vi "getSparaConfig.vi"(0 "Spec Associate":string[][](table), 5 "different":string[](array[string]), 9 "smooth":bool[](array[boolean]), 11 "XML document":path caption="XML文档路径", 12 "smoothPoints":dbl=1.0 min=1.0 max=100.0 step=2.0) -> (4 "sPara":T1[](array[typedef]), 6 "extPara":T1[](array[typedef]))   [LabVIEW 2011]
uses:
  dataType/singleTestParameter.ctl
panel:
  out "extParaSmooth":bool[](array[boolean])
  out "sParaSmooth":bool[](array[boolean])
  in  "spec 2":T2
  in  "spec":T2
  out "namelist":string[](array[string])
  out "valueArray":string[][](array[string])
  out "extPara":string[](array[string])
  out "sPara":string[](array[string])
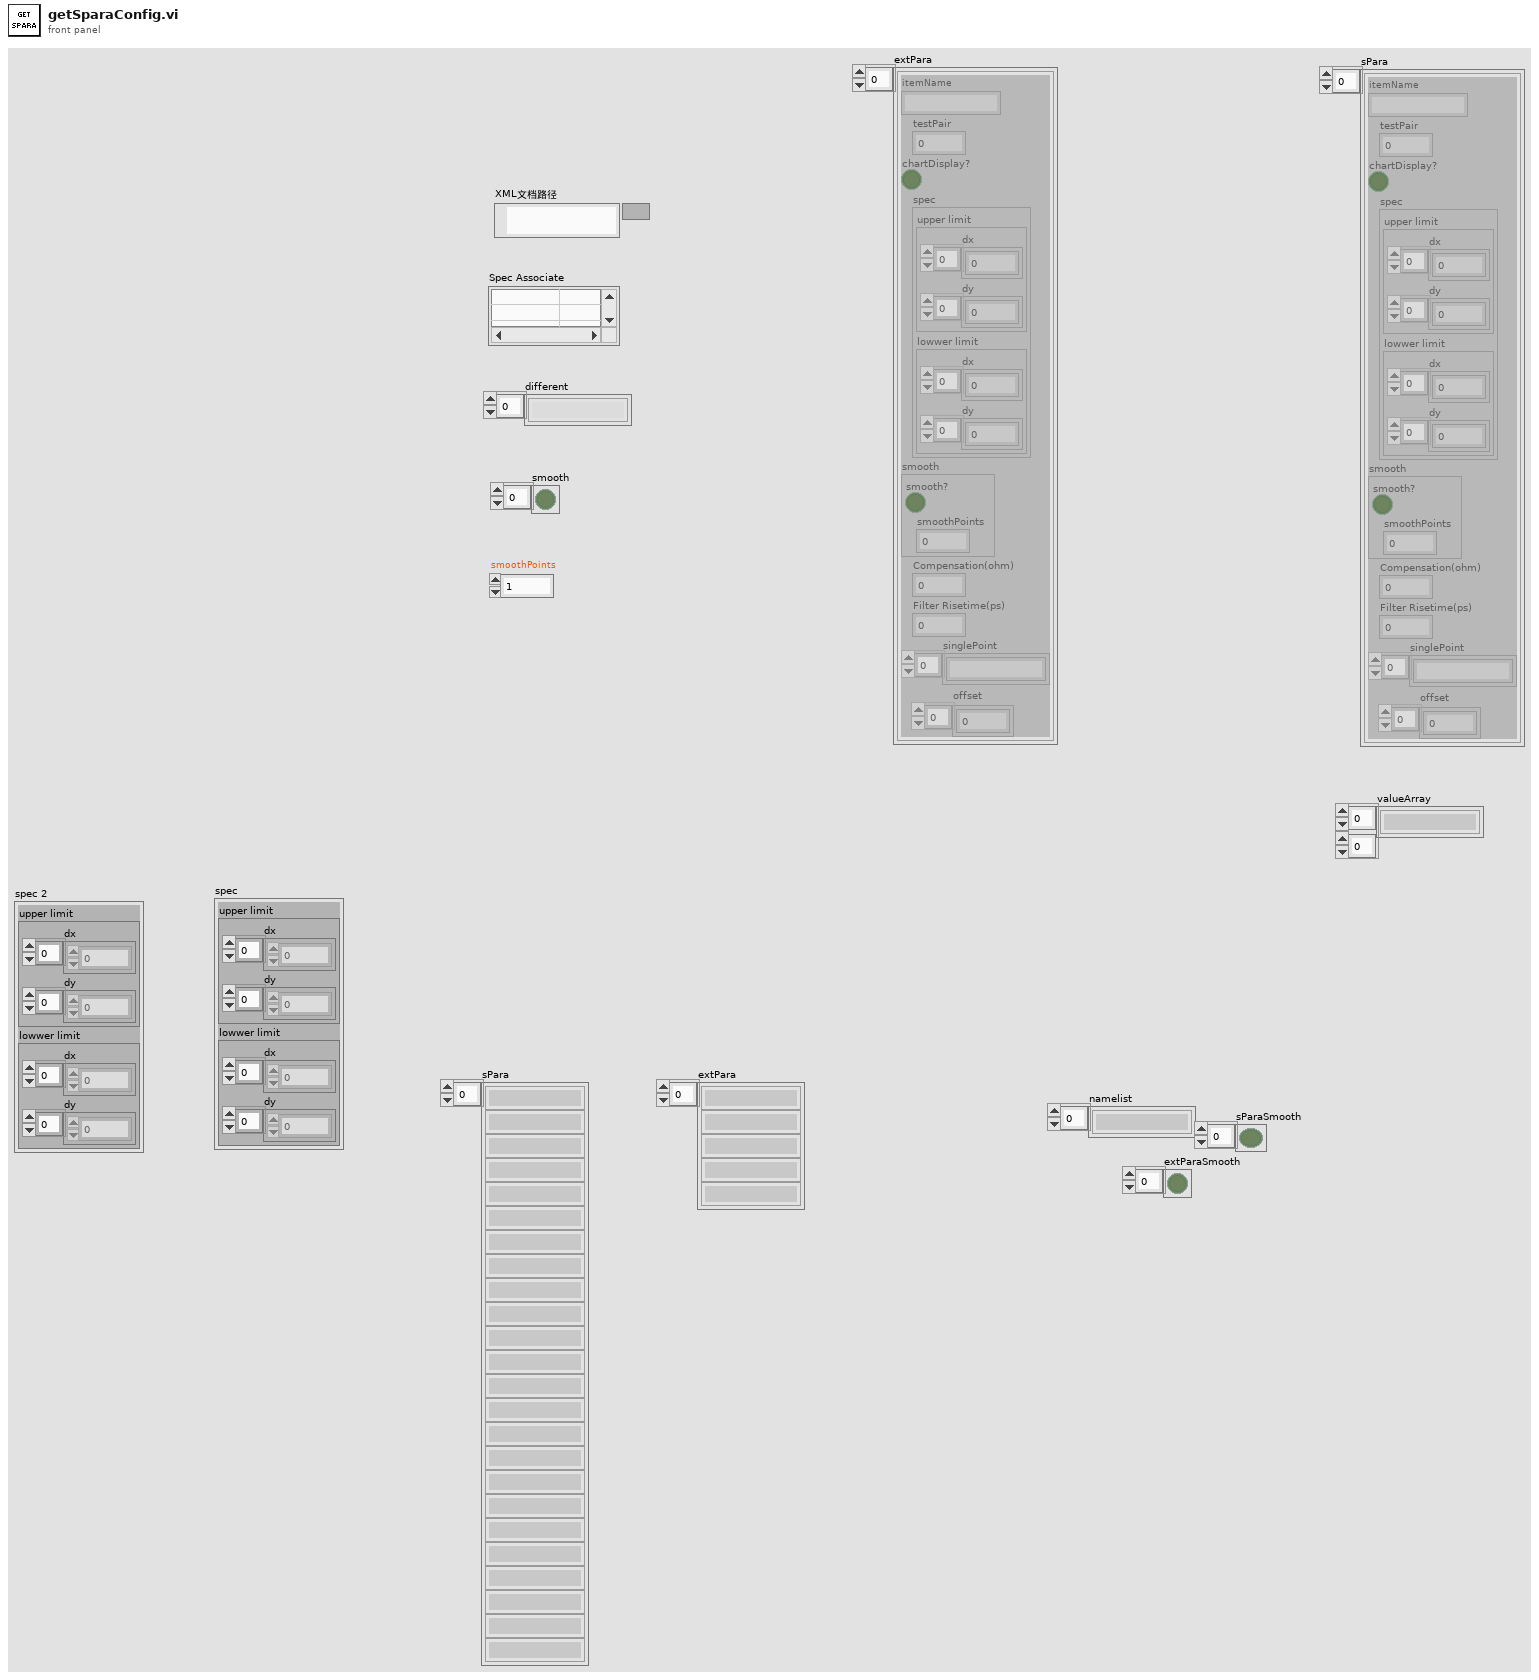
[diagram p1: front panel]
types:
  T1 = typedef "singleTestParameter.ctl" = cluster{"itemName":string, "testPair":dbl, "chartDisplay?":bool, "spec":cluster{"upper limit":cluster{"dx":dbl[], "dy":dbl[]}, "lowwer limit":cluster{"dx":dbl[], "dy":dbl[]}}, "smooth":cluster{"smooth?":bool, "smoothPoints":dbl}, "Compensation(ohm)":dbl, "Filter Risetime(ps)":dbl, "singlePoint":string[], "offset":dbl[]}
  T2 = cluster{"upper limit":cluster{"dx":dbl[], "dy":dbl[]}, "lowwer limit":cluster{"dx":dbl[], "dy":dbl[]}}
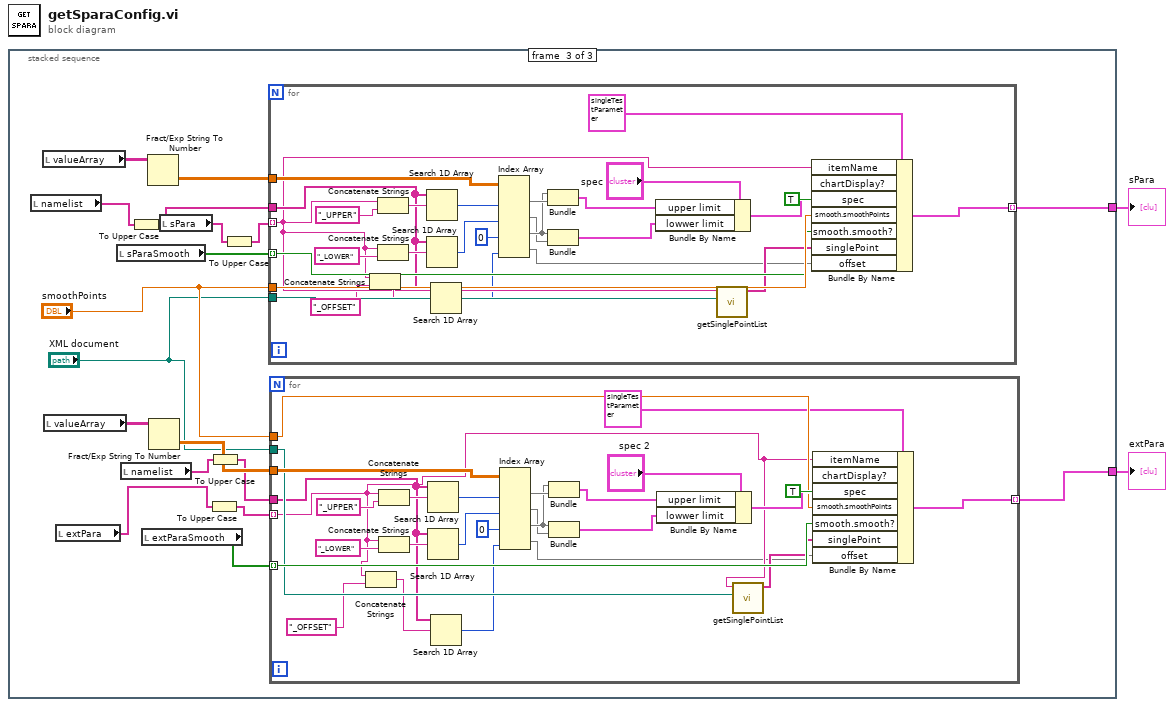
[diagram p0: block diagram]
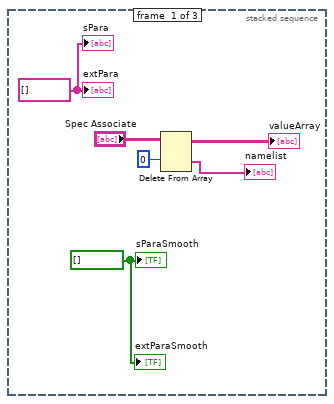
[diagram p2: hidden frame]
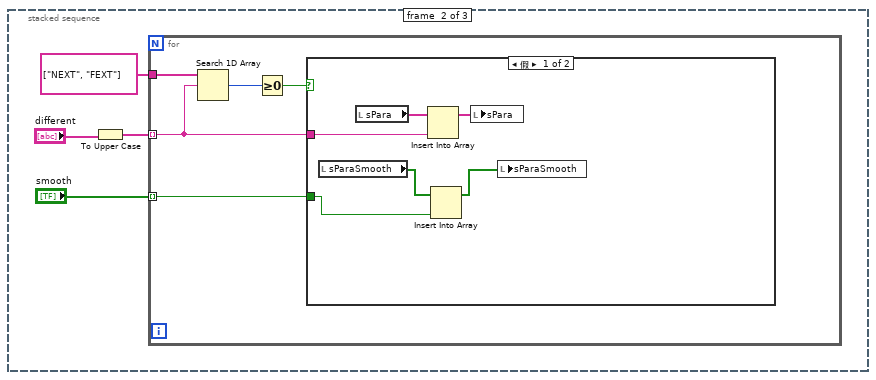
[diagram p3: hidden frame]
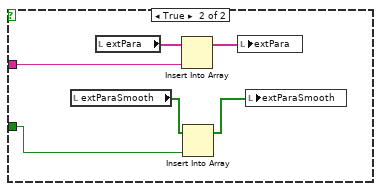
[diagram p4: hidden frame]
diagram:
  n1 = stacked-sequence {
    tunnel: [_ _ w43] -> w2
    tunnel: [_ _ w42] -> w1
    frame #0 {
      w3 = bool[] []
      w8 = string[] [] ("数组")
      n2 = Delete From Array(array="Spec Associate", index (row)=0 ("索引 (行)")) -> (deleted portion=→"namelist":string[], array with subset deleted=→"valueArray":string[][])  [unwired: 2 in]
      "sPara" <- w8
      "extPara" <- w8
      "sParaSmooth" <- w3
      "extParaSmooth" <- w3
    }
    frame #1 {
      n3 = To Upper Case(1:"different") -> (0:w11:string[])
      n4 = for {
        tunnel: w11 -> [w16] mode=indexing
        tunnel: string[] ["NEXT", "FEXT"] -> [w17]
        tunnel: "smooth" -> [w13] mode=indexing
        n5 = Search 1D Array(1D array=w17, element=w16) -> (index of element=w15:i32)  [unwired: 1 in]
        n6 = Greater Or Equal To 0?(x=w15) -> (x >= 0?=w14:bool)
        n7 = case shown="假" w14 {
          tunnel: w16 -> [w21 w29]
          tunnel: w13 -> [w18 w24]
          frame False {
            n8 = local read "sParaSmooth"() -> (w19:bool[])
            n9 = local read "sPara"() -> (w23:string[])
            n10 = Insert Into Array(array=w23, new element=w21) -> (w22:string[])  [unwired: 1 in]
            n11 = Insert Into Array(array=w19, new element=w18) -> (w20:bool[])  [unwired: 1 in]
            n12 = local write "sPara"(w22) -> ()
            n13 = local write "sParaSmooth"(w20) -> ()
          }
          frame True {
            n14 = local read "extParaSmooth"() -> (w25:bool[])
            n15 = local read "extPara"() -> (w28:string[])
            n16 = Insert Into Array(array=w28, new element=w29) -> (w27:string[])  [unwired: 1 in]
            n17 = Insert Into Array(array=w25, new element=w24) -> (w26:bool[])  [unwired: 1 in]
            n18 = local write "extPara"(w27) -> ()
            n19 = local write "extParaSmooth"(w26) -> ()
          }
        }
      }
    }
    frame #2 {
      n20 = local read "namelist"() -> (w38:string[])
      n21 = local read "valueArray"() -> (w47:string[][])
      n22 = local read "valueArray"() -> (w45:string[][])
      n23 = local read "extPara"() -> (w34:string[])
      n24 = local read "sParaSmooth"() -> (w40:bool[])
      n25 = local read "namelist"() -> (w36:string[])
      n26 = To Upper Case(1:w38) -> (0:w37:string[])
      n27 = local read "extParaSmooth"() -> (w39:bool[])
      n28 = Fract/Exp String To Number(string=w47) -> (number=w46:dbl[][])  [unwired: 3 in, 1 out]
      n29 = Fract/Exp String To Number(string=w45) -> (number=w44:dbl[][])  [unwired: 3 in, 1 out]
      n30 = local read "sPara"() -> (w32:string[])
      n31 = To Upper Case(1:w34) -> (0:w33:string[])
      n32 = To Upper Case(1:w36) -> (0:w35:string[])
      n33 = To Upper Case(1:w32) -> (0:w31:string[])
      n34 = for {
        tunnel: w31 -> [w79] mode=indexing
        tunnel: w37 -> [w81]
        tunnel: w46 -> [w98]
        tunnel: [w87] -> w43 mode=indexing
        tunnel: "smoothPoints" -> [w86]
        tunnel: w40 -> [w85] mode=indexing
        tunnel: "XML document" -> [w83]
        n35 = Concatenate Strings(w79, "_OFFSET" ("字符串")) -> (w80:string)
        n36 = Concatenate Strings(w79, "_UPPER" ("字符串")) -> (w101:string)
        n37 = Concatenate Strings(w79, "_LOWER" ("字符串")) -> (w99:string)
        n38 = Search 1D Array(1D array=w81, element=w101) -> (index of element=w97:i32)  [unwired: 1 in]
        n39 = Search 1D Array(1D array=w81, element=w99) -> (index of element=w96:i32)  [unwired: 1 in]
        n40 = Search 1D Array(1D array=w81, element=w80) -> (index of element=w77:i32)  [unwired: 1 in]
        n41 = Index Array(array=w98, index (col) #1=w97, index (col) #2=w96, index (col) #3=0 ("索引 (列)"), index (col) #4=w77) -> (element #1=w94:dbl[], element #2=w91:dbl[], element #3=w92:dbl[], element #4=w76:dbl[])  [unwired: 4 in]
        n42 = Bundle(w92, w94) -> (w93:cluster{dbl[], dbl[]})  [unwired: 1 in]
        n43 = Bundle(w92, w91) -> (w90:cluster{dbl[], dbl[]})  [unwired: 1 in]
        n44 = Bundle By Name(cluster="spec", "upper limit"=w93, "lowwer limit"=w90) -> (w88:T2)
        n45 = call "getSinglePointList.vi"("XML document"=w83, "itemName"=w79) -> ("pointList"=w82:string[])  [unwired: 9 in]
        n46 = Bundle By Name(cluster=T1 {"itemName"="", "testPair"=0.0, "chartDisplay?"=FALSE, "spec"={"upper limit"={"dx"=[], "dy"=[]}, "lowwer limit"={"dx"=[], "dy"=[]}}, "smooth"={"smooth?"=FALSE, "smoothPoints"=0.0}, "Compensation(ohm)"=0.0, "Filter Risetime(ps)"=0.0, "singlePoint"=[], "offset"=[]} ("singleTestParameter"), "itemName"=w79, "chartDisplay?"=TRUE, "spec"=w88, "smooth.smoothPoints"=w86, "smooth.smooth?"=w85, "singlePoint"=w82, "offset"=w76) -> (w87:T1)
      }
      n47 = for {
        tunnel: w33 -> [w51] mode=indexing
        tunnel: w35 -> [w53]
        tunnel: w44 -> [w70]
        tunnel: [w59] -> w42 mode=indexing
        tunnel: "smoothPoints" -> [w58]
        tunnel: w39 -> [w57] mode=indexing
        tunnel: "XML document" -> [w54]
        n48 = Concatenate Strings(w51, "_OFFSET" ("字符串")) -> (w52:string)
        n49 = Concatenate Strings(w51, "_UPPER" ("字符串")) -> (w73:string)
        n50 = Concatenate Strings(w51, "_LOWER" ("字符串")) -> (w71:string)
        n51 = Search 1D Array(1D array=w53, element=w73) -> (index of element=w69:i32)  [unwired: 1 in]
        n52 = Search 1D Array(1D array=w53, element=w71) -> (index of element=w68:i32)  [unwired: 1 in]
        n53 = Search 1D Array(1D array=w53, element=w52) -> (index of element=w49:i32)  [unwired: 1 in]
        n54 = Index Array(array=w70, index (col) #1=w69, index (col) #2=w68, index (col) #3=0 ("索引 (列)"), index (col) #4=w49) -> (element #1=w66:dbl[], element #2=w63:dbl[], element #3=w64:dbl[], element #4=w48:dbl[])  [unwired: 4 in]
        n55 = Bundle(w64, w66) -> (w65:cluster{dbl[], dbl[]})  [unwired: 1 in]
        n56 = Bundle(w64, w63) -> (w62:cluster{dbl[], dbl[]})  [unwired: 1 in]
        n57 = Bundle By Name(cluster="spec 2", "upper limit"=w65, "lowwer limit"=w62) -> (w60:T2)
        n58 = call "getSinglePointList.vi"("XML document"=w54, "itemName"=w51) -> ("pointList"=w55:string[])  [unwired: 9 in]
        n59 = Bundle By Name(cluster=T1 {"itemName"="", "testPair"=0.0, "chartDisplay?"=FALSE, "spec"={"upper limit"={"dx"=[], "dy"=[]}, "lowwer limit"={"dx"=[], "dy"=[]}}, "smooth"={"smooth?"=FALSE, "smoothPoints"=0.0}, "Compensation(ohm)"=0.0, "Filter Risetime(ps)"=0.0, "singlePoint"=[], "offset"=[]} ("singleTestParameter"), "itemName"=w51, "chartDisplay?"=TRUE, "spec"=w60, "smooth.smoothPoints"=w58, "smooth.smooth?"=w57, "singlePoint"=w55, "offset"=w48) -> (w59:T1)
      }
    }
  }
  "sPara" <- w2
  "extPara" <- w1
